vi "CloseErrorFile.vi"(5 "Error In":errorcluster) -> (19 "Error Out":errorcluster)   [LabVIEW 2018, in "Error handler.lvclass"]
uses:
  Error handler.lvclass
  ErrorLogFile_class/ErrorLogFile.lvclass
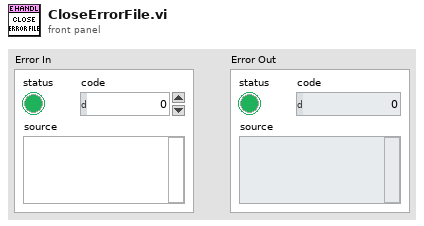
[diagram p1: front panel]
types:
  T1 = typedef "Error handler.lvclass/ObjectAttributes.ctl" = cluster{"ErrorBroadcastEvent":refnum<user-event>, "LoadFPOnError":bool, "ErrorLogFile":refnum<class "ErrorLogFile.lvclass">, "Testing":bool, "Name":string}
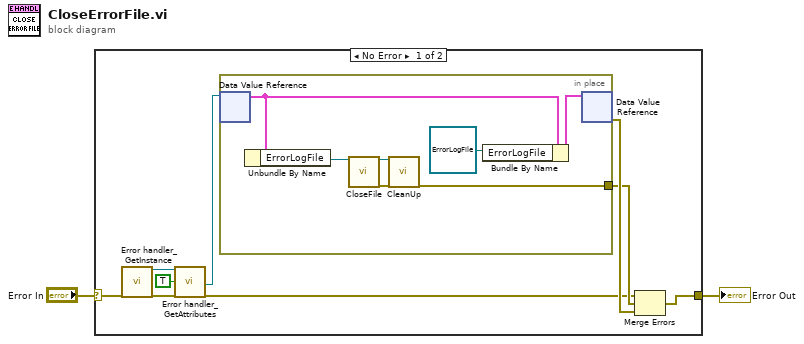
[diagram p0: block diagram]
diagram:
  n1 = case shown="No Error" "Error In" {
    selector: "Error In" -> [w9 w19]
    tunnel: [w3 w19] -> w1
    frame No Error {
      n2 = call "Error handler_GetInstance.vi"("error in"=w9) -> ("reference out"=w11:refnum<class "Error handler.lvclass">, "error out"=w10:errorcluster)  [unwired: 14 in, 3 out]
      n3 = call "Error handler_GetAttributes.vi"("reference in"=w11, "OnlyGetDvrReference(False)"=TRUE, "error in (no error)"=w10) -> ("DataRef"=w6:refnum<data-value>, "error out"=w4:errorcluster)  [unwired: 13 in, 2 out]
      n4 = in-place {
        in-place-border: [w12] -> w5
        n5 = in-place-dvr #1(w6) -> (w16:T1)  [unwired: 1 out]
        n6 = Unbundle By Name(w16) -> ("ErrorLogFile"=w15:refnum<class "ErrorLogFile.lvclass">)
        n7 = call-dynamic "CloseFile.vi"("object in"=w15) -> ("object out"=w13:refnum<class "ErrorLogFile.lvclass">, "Error Out"=w14:errorcluster)  [unwired: 17 in]
        n8 = call-dynamic "CleanUp.vi"("object in"=w13, "Error In"=w14) -> ("Error Out"=w12:errorcluster)  [unwired: 17 in]
        n9 = Bundle By Name(cluster=w16, "ErrorLogFile"=refnum<class "ErrorLogFile.lvclass"> refnum) -> (w18:T1)
        n10 = in-place-dvr #1(w18) -> (w7:errorcluster)  [unwired: 1 out]
      }
      n11 = Merge Errors(w4, w5, w7) -> (w3:errorcluster)
    }
    frame Error {
    }
  }
  "Error Out" <- w1
